vi "Check Password (SubVI).vi"(8 "error in (no error)":errorcluster, 11 "trimmed string":string) -> (0 "error out":errorcluster, 3 "Checkbox":bool)   [LabVIEW 2020, in "Notification.lvlib"]
uses:
  Notification.lvlib
  <vilib>/Utility/config.llb/Read Key (String).vi
  <vilib>/Utility/config.llb/NI_LVConfig.lvlib
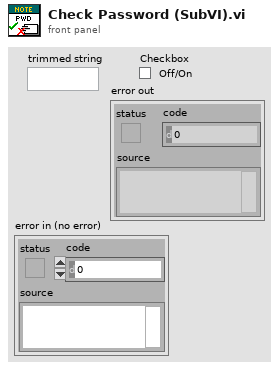
[diagram p1: front panel]
types:
  T1 = typedef "NI_LVConfig.lvlib/Config Data RefNum.ctl" = refnum<k1>
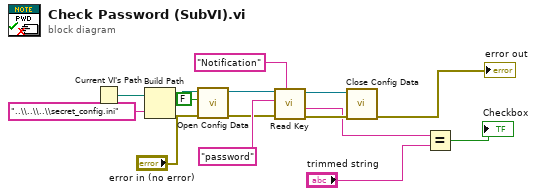
[diagram p0: block diagram]
diagram:
  n1 = Current VI's Path() -> (path=w13:path)
  n2 = Build Path(base path=w13, name or relative path="..\\..\\..\\secret_config.ini") -> (appended path=w11:path)
  n3 = call <vilib>:"Open Config Data.vi"("error in (no error)"="error in (no error)", "create file if necessary (T)"=FALSE, "configuration file path"=w11) -> ("error out"=w6:errorcluster, "refnum"=w10:T1)  [unwired: 6 in, 1 out]
  n4 = call-poly <vilib>:"Read Key.vi"("section"="Notification", "error in (no error)"=w6, "key"="password", "refnum"=w10) -> ("error out"=w5:errorcluster, "value"=w4:string, "refnum out"=w9:T1)  [unwired: 4 in, 1 out]
  n5 = call <vilib>:"Close Config Data.vi"("error in (no error)"=w5, "refnum"=w9) -> ("error out"=→"error out":errorcluster)  [unwired: 8 in, 1 out]
  n6 = Equal?(x=w4, y="trimmed string") -> (x = y?=→"Checkbox":bool)
